vi "Add Property (Cluster).vi"(7 "required?":bool, 8 "error in (no error)":errorcluster, 9 "root level? (false)":bool, 10 "Cluster in":refnum<vi>, 11 "JSON Schema in":string) -> (0 "error out":errorcluster, 3 "JSON Schema out":string)   [LabVIEW 2020, in "JSON Schema Generator.lvlib"]
uses:
  JSON Schema Generator.lvlib
  <vilib>/JDP Science/JSONtext/JSONtext.lvlib
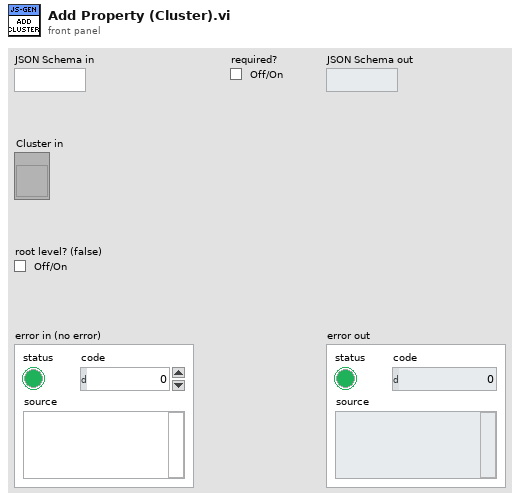
[diagram p1: front panel]
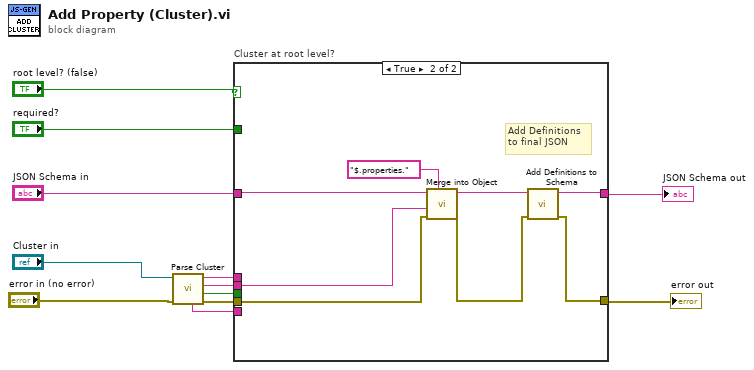
[diagram p0: block diagram]
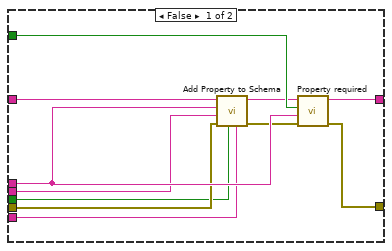
[diagram p2: hidden frame]
diagram:
  n1 = call "Parse Cluster.vi"("error in"="error in (no error)", "Cluster Refnum In"="Cluster in") -> ("error out"=w5:errorcluster, "Typedef?"=w2:bool, "JSON ObjectSchema out"=w9:string, "JSON Object Name"=w12:string, "Typedef Name"=w1:string)  [unwired: 5 in]
  n2 = case "Cluster at root level?" shown="True" "root level? (false)" {
    tunnel: w12 -> [w18 _]
    tunnel: "required?" -> [w23 _]
    tunnel: [w22 w27] -> w10
    tunnel: w9 -> [w17 w29]
    tunnel: "JSON Schema in" -> [w20 w30]
    tunnel: w5 -> [w16 w24]
    tunnel: [w21 w25] -> w4
    tunnel: w2 -> [w14 _]
    tunnel: w1 -> [w13 _]
    frame False {
      n3 = call "Add Property to Schema.vi"("Typedef Name"=w13, "Typedef?"=w14, "error in"=w16, "JSON Schema Property in"=w17, "Property Name"=w18, "JSON Schema in"=w20) -> ("error out"=w15:errorcluster, "JSON Schema out"=w19:string)  [unwired: 4 in]
      n4 = call "Property required.vi"("error in (no error)"=w15, "Name"=w18, "Required?"=w23, "JSON Schema in"=w19) -> ("error out"=w21:errorcluster, "JSON Schema out"=w22:string)  [unwired: 6 in]
    }
    frame True {
      # "Add Definitions\nto final JSON"
      n5 = call <vilib>:"Merge into Object.vi"("$Path or Item Name"="$.properties.", "error in (no error)"=w24, "JSON Object to Merge"=w29, "JSON"=w30) -> ("error out"=w26:errorcluster, "<JSON>"=w28:string)  [unwired: 5 in]
      n6 = call "Add Definitions to Schema.vi"("error in (no error)"=w26, "JSON In"=w28) -> ("error out"=w25:errorcluster, "JSON Out"=w27:string)  [unwired: 8 in]
    }
  }
  "JSON Schema out" <- w10
  "error out" <- w4
